vi "从数据库获取数据通用可配置(子VI).vi"(8 "错误输入（无错误）":errorcluster, 9 "查询参数数组":string[](array[string])=["CODMn", "CODCr", "DO", "铜", "PH", "氨氮", "比电导率", "水温", "COD", "浊度", "总氮", "总磷", "叶绿素a", "藻密度", "水位", "流速", "瞬时流量", "累积流量", "亚硝酸盐", "硫化物", "ORP", "铅", "镉", "锌", "镍", "锰", "汞"], 10 "table输入":string="实时数据") -> (0 "错误输出":errorcluster, 3 "簇数组":cluster{"待发送数据":string[][]}[][](array[cluster]))   [LabVIEW 2016, in "数据传输系统-02.lvlib"]
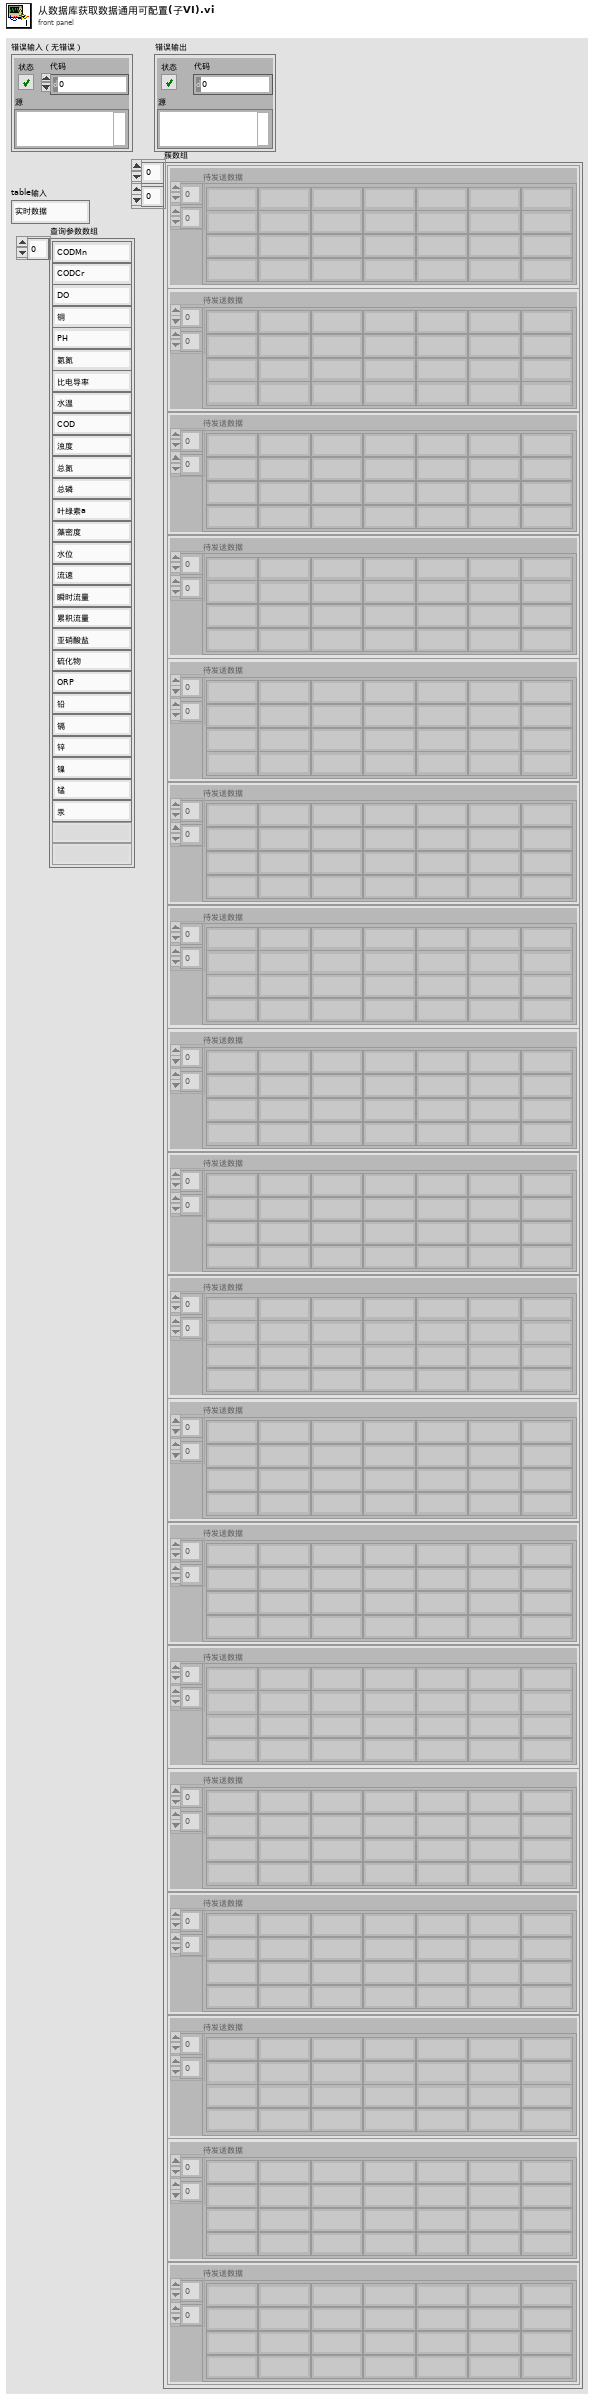
[diagram p1: front panel]
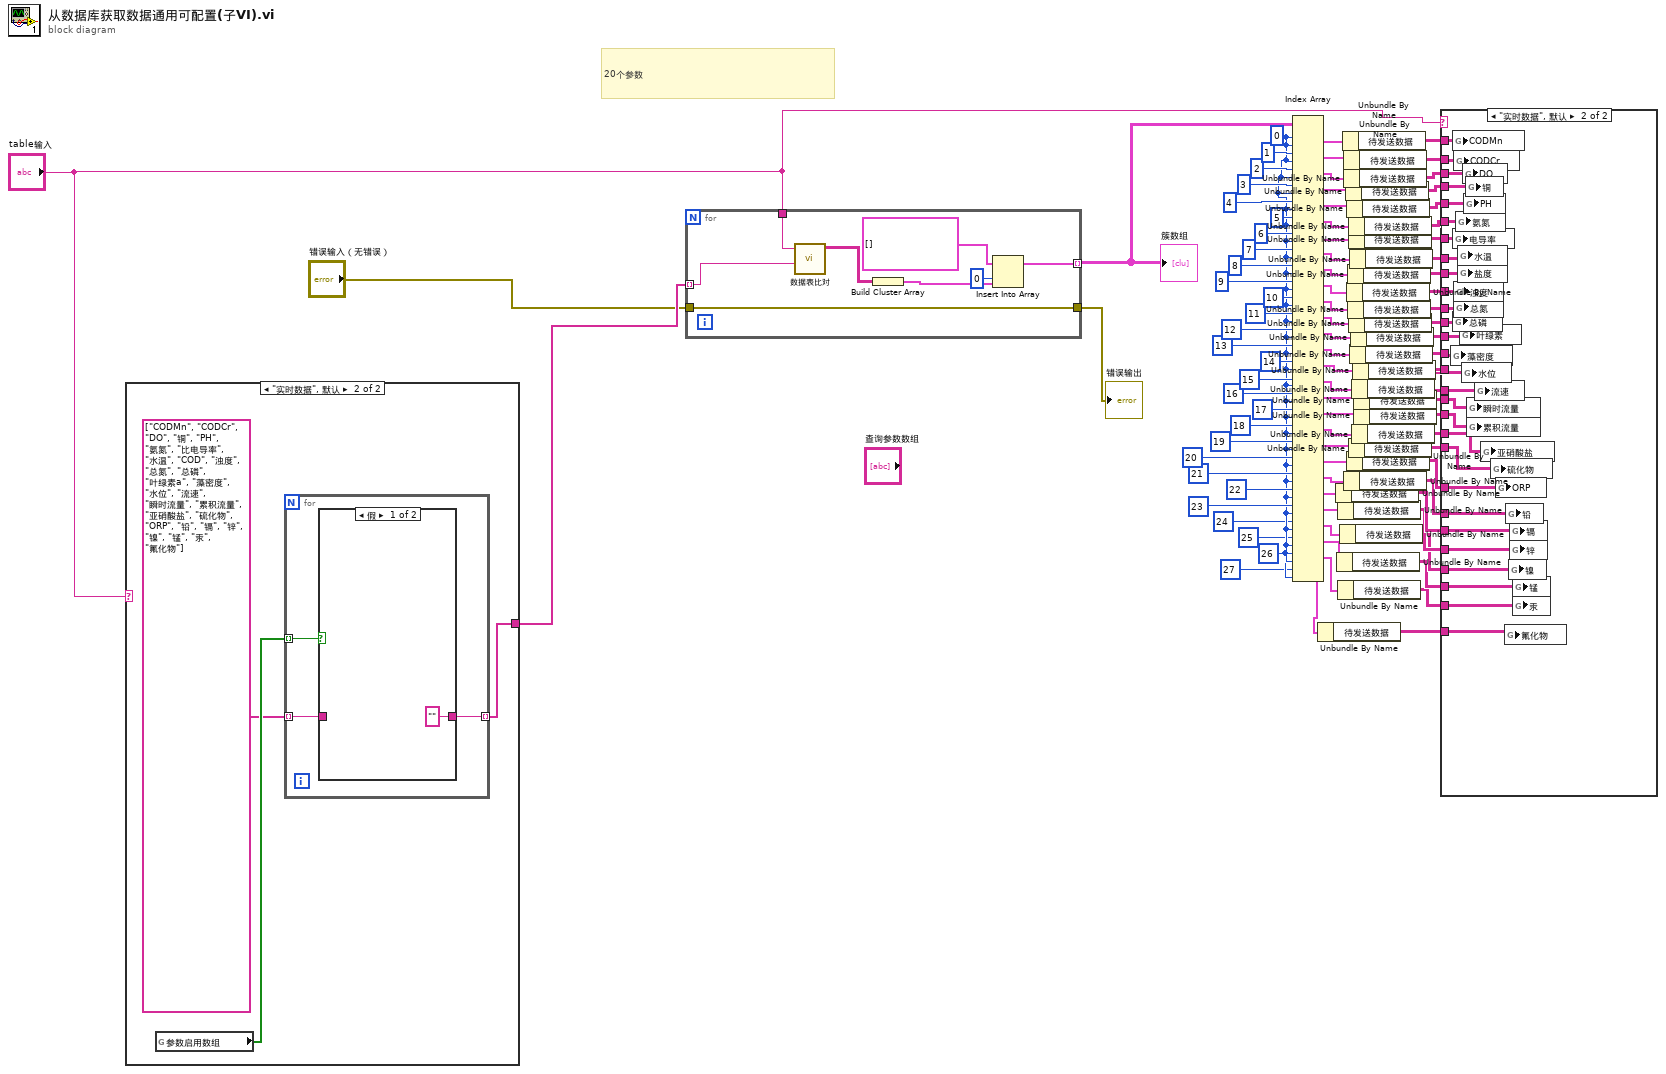
[diagram p0: block diagram]
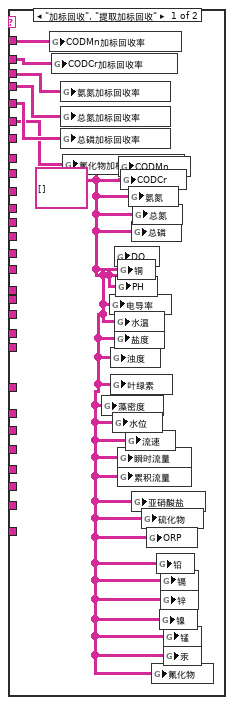
[diagram p2: hidden frame]
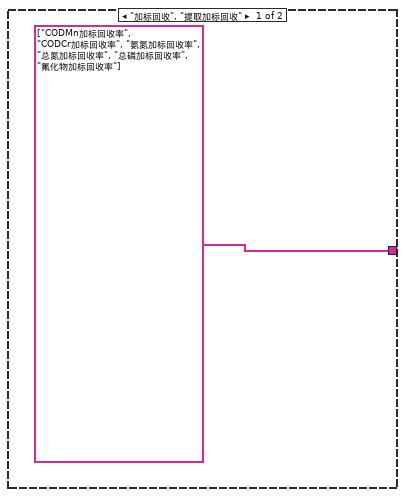
[diagram p3: hidden frame]
diagram:
  w4 = 26 ("禁用的索引 (行)")
  w14 = 0 ("索引 (行)")
  # "20个参数"
  n1 = case shown="\"实时数据\", 默认" "table输入" {
    tunnel: [string[] ["CODMn加标回收率", "CODCr加标回收率", "氨氮加标回收率", "总氮加标回收率", "总磷加标回收率", "氟化物加标回收率"] ("查询参数数组") w91] -> w46
    frame "加标回收", "提取加标回收" {
    }
    frame "实时数据", Default {
      n2 = global read "断电保存全局.vi" "参数启用数组"() -> (w93:bool[])
      n3 = for {
        tunnel: w93 -> [w96] mode=indexing
        tunnel: string[] ["CODMn", "CODCr", "DO", "铜", "PH", "氨氮", "比电导率", "水温", "COD", "浊度", "总氮", "总磷", "叶绿素a", "藻密度", "水位", "流速", "瞬时流量", "累积流量", "亚硝酸盐", "硫化物", "ORP", "铅", "镉", "锌", "镍", "锰", "汞", "氟化物"] ("数组") -> [w95] mode=indexing
        tunnel: [w94] -> w91 mode=indexing
        n4 = case shown="假" w96 {
          tunnel: ["" w98] -> w94
          tunnel: w95 -> [_ w98]
          frame False {
          }
          frame True {
          }
        }
      }
    }
  }
  n5 = for {
    tunnel: w46 -> [w100] mode=indexing
    tunnel: [w104] -> w88 mode=indexing
    tunnel: "table输入" -> [w101]
    tunnel: [w99] -> w89
    tunnel: "错误输入（无错误）" -> [w99]
    n6 = call "数据表比对.vi"("查询元素输入"=w100, "table输入"=w101) -> ("待发送数据"=w106:string[][])  [unwired: 6 in, 3 out]
    n7 = Build Cluster Array(w106) -> (w105:cluster{"待发送数据":string[][]}[])
    n8 = Insert Into Array(array=cluster{"待发送数据":string[][]}[] [] ("簇数组"), index=0 ("索引"), new element=w105) -> (w104:cluster{"待发送数据":string[][]}[])
  }
  "簇数组" <- w88
  "错误输出" <- w89
  n9 = Index Array(array=w88, index (row) #1=w14, index (col) #1=w14, index (row) #2=1 ("索引 (行)"), index (col) #2=w14, index (row) #3=2 ("索引 (行)"), index (col) #3=w14, index (row) #4=3 ("索引 (行)"), index (col) #4=w14, index (row) #5=4 ("索引 (行)"), index (col) #5=w14, index (row) #6=5 ("索引 (行)"), index (col) #6=w14, index (row) #7=6 ("索引 (行)"), index (col) #7=w14, index (row) #8=7 ("索引 (行)"), index (col) #8=w14, index (row) #9=8 ("索引 (行)"), index (col) #9=w14, index (row) #10=9 ("索引 (行)"), index (col) #10=w14, index (row) #11=10 ("索引 (行)"), index (col) #11=w14, index (row) #12=11 ("索引 (行)"), index (col) #12=w14, index (row) #13=12 ("索引 (行)"), index (col) #13=w14, index (row) #14=13 ("索引 (行)"), index (col) #14=w14, index (row) #15=14 ("禁用的索引 (行)"), index (col) #15=w14, index (row) #16=15 ("禁用的索引 (行)"), index (col) #16=w14, index (row) #17=16 ("禁用的索引 (行)"), index (col) #17=w14, index (row) #18=17 ("禁用的索引 (行)"), index (col) #18=w14, index (row) #19=18 ("禁用的索引 (行)"), index (col) #19=w14, index (row) #20=19 ("禁用的索引 (行)"), index (col) #20=w14, index (row) #21=20 ("禁用的索引 (行)"), index (col) #21=w14, index (row) #22=21 ("禁用的索引 (行)"), index (col) #22=w14, index (row) #23=22 ("禁用的索引 (行)"), index (col) #23=w14, index (row) #24=23 ("禁用的索引 (行)"), index (col) #24=w14, index (row) #25=24 ("禁用的索引 (行)"), index (col) #25=w14, index (row) #26=25 ("禁用的索引 (行)"), index (col) #26=w14, index (row) #27=w4, index (col) #27=w14, index (row) #28=27 ("禁用的索引 (行)"), index (col) #28=w4) -> (element #1=w87:cluster{"待发送数据":string[][]}, element #2=w72:cluster{"待发送数据":string[][]}, element #3=w71:cluster{"待发送数据":string[][]}, element #4=w70:cluster{"待发送数据":string[][]}, element #5=w69:cluster{"待发送数据":string[][]}, element #6=w68:cluster{"待发送数据":string[][]}, element #7=w66:cluster{"待发送数据":string[][]}, element #8=w67:cluster{"待发送数据":string[][]}, element #9=w65:cluster{"待发送数据":string[][]}, element #10=w64:cluster{"待发送数据":string[][]}, element #11=w63:cluster{"待发送数据":string[][]}, element #12=w62:cluster{"待发送数据":string[][]}, element #13=w61:cluster{"待发送数据":string[][]}, element #14=w60:cluster{"待发送数据":string[][]}, element #15=w41:cluster{"待发送数据":string[][]}, element #16=w39:cluster{"待发送数据":string[][]}, element #17=w38:cluster{"待发送数据":string[][]}, element #18=w37:cluster{"待发送数据":string[][]}, element #19=w32:cluster{"待发送数据":string[][]}, element #20=w28:cluster{"待发送数据":string[][]}, element #21=w27:cluster{"待发送数据":string[][]}, element #22=w20:cluster{"待发送数据":string[][]}, element #23=w19:cluster{"待发送数据":string[][]}, element #24=w18:cluster{"待发送数据":string[][]}, element #25=w11:cluster{"待发送数据":string[][]}, element #26=w9:cluster{"待发送数据":string[][]}, element #27=w8:cluster{"待发送数据":string[][]}, element #28=w2:cluster{"待发送数据":string[][]})
  n10 = Unbundle By Name(w2) -> ("待发送数据"=w1:string[][])
  n11 = Unbundle By Name(w19) -> ("待发送数据"=w16:string[][])
  n12 = Unbundle By Name(w9) -> ("待发送数据"=w7:string[][])
  n13 = Unbundle By Name(w18) -> ("待发送数据"=w15:string[][])
  n14 = Unbundle By Name(w8) -> ("待发送数据"=w6:string[][])
  n15 = Unbundle By Name(w11) -> ("待发送数据"=w10:string[][])
  n16 = Unbundle By Name(w87) -> ("待发送数据"=w86:string[][])
  n17 = Unbundle By Name(w72) -> ("待发送数据"=w59:string[][])
  n18 = Unbundle By Name(w71) -> ("待发送数据"=w58:string[][])
  n19 = Unbundle By Name(w20) -> ("待发送数据"=w17:string[][])
  n20 = Unbundle By Name(w70) -> ("待发送数据"=w57:string[][])
  n21 = Unbundle By Name(w69) -> ("待发送数据"=w56:string[][])
  n22 = Unbundle By Name(w64) -> ("待发送数据"=w51:string[][])
  n23 = Unbundle By Name(w27) -> ("待发送数据"=w24:string[][])
  n24 = Unbundle By Name(w65) -> ("待发送数据"=w52:string[][])
  n25 = Unbundle By Name(w63) -> ("待发送数据"=w50:string[][])
  n26 = Unbundle By Name(w68) -> ("待发送数据"=w55:string[][])
  n27 = Unbundle By Name(w66) -> ("待发送数据"=w54:string[][])
  n28 = Unbundle By Name(w62) -> ("待发送数据"=w49:string[][])
  n29 = Unbundle By Name(w28) -> ("待发送数据"=w25:string[][])
  n30 = Unbundle By Name(w67) -> ("待发送数据"=w53:string[][])
  n31 = Unbundle By Name(w60) -> ("待发送数据"=w48:string[][])
  n32 = Unbundle By Name(w61) -> ("待发送数据"=w47:string[][])
  n33 = Unbundle By Name(w39) -> ("待发送数据"=w36:string[][])
  n34 = Unbundle By Name(w32) -> ("待发送数据"=w26:string[][])
  n35 = Unbundle By Name(w41) -> ("待发送数据"=w40:string[][])
  n36 = Unbundle By Name(w38) -> ("待发送数据"=w35:string[][])
  n37 = Unbundle By Name(w37) -> ("待发送数据"=w34:string[][])
  n38 = case shown="\"实时数据\", 默认" "table输入" {
    tunnel: w86 -> [w113 w141]
    tunnel: w59 -> [w112 w140]
    tunnel: w58 -> [w111 w139]
    tunnel: w57 -> [w110 w138]
    tunnel: w56 -> [w109 w137]
    tunnel: w55 -> [w108 w136]
    tunnel: w54 -> [_ w135]
    tunnel: w53 -> [_ w134]
    tunnel: w52 -> [_ w133]
    tunnel: w51 -> [_ w132]
    tunnel: w50 -> [_ w131]
    tunnel: w49 -> [_ w130]
    tunnel: w48 -> [_ w129]
    tunnel: w47 -> [_ w128]
    tunnel: w40 -> [_ w127]
    tunnel: w36 -> [_ w126]
    tunnel: w35 -> [_ w125]
    tunnel: w34 -> [_ w124]
    tunnel: w26 -> [_ w123]
    tunnel: w25 -> [_ w122]
    tunnel: w24 -> [_ w121]
    tunnel: w17 -> [_ w120]
    tunnel: w16 -> [_ w119]
    tunnel: w15 -> [_ w118]
    tunnel: w10 -> [_ w117]
    tunnel: w7 -> [_ w116]
    tunnel: w6 -> [_ w115]
    tunnel: w1 -> [_ w114]
    frame "加标回收", "提取加标回收" {
      w107 = string[][] [] ("DO")
      n39 = global write "全局 所有参数.vi" "CODMn加标回收率"(w113) -> ()
      n40 = global write "全局 所有参数.vi" "CODCr加标回收率"(w112) -> ()
      n41 = global write "全局 所有参数.vi" "氨氮加标回收率"(w111) -> ()
      n42 = global write "全局 所有参数.vi" "总氮加标回收率"(w110) -> ()
      n43 = global write "全局 所有参数.vi" "总磷加标回收率"(w109) -> ()
      n44 = global write "全局 所有参数.vi" "氟化物加标回收率"(w108) -> ()
      n45 = global write "全局 所有参数.vi" "藻密度"(w107) -> ()
      n46 = global write "全局 所有参数.vi" "电导率"(w107) -> ()
      n47 = global write "全局 所有参数.vi" "浊度"(w107) -> ()
      n48 = global write "全局 所有参数.vi" "叶绿素"(w107) -> ()
      n49 = global write "全局 所有参数.vi" "水位"(w107) -> ()
      n50 = global write "全局 所有参数.vi" "DO"(w107) -> ()
      n51 = global write "全局 所有参数.vi" "水温"(w107) -> ()
      n52 = global write "全局 所有参数.vi" "盐度"(w107) -> ()
      n53 = global write "全局 所有参数.vi" "PH"(w107) -> ()
      n54 = global write "全局 所有参数.vi" "铜"(w107) -> ()
      n55 = global write "全局 所有参数.vi" "瞬时流量"(w107) -> ()
      n56 = global write "全局 所有参数.vi" "累积流量"(w107) -> ()
      n57 = global write "全局 所有参数.vi" "CODMn"(w107) -> ()
      n58 = global write "全局 所有参数.vi" "CODCr"(w107) -> ()
      n59 = global write "全局 所有参数.vi" "流速"(w107) -> ()
      n60 = global write "全局 所有参数.vi" "氨氮"(w107) -> ()
      n61 = global write "全局 所有参数.vi" "总磷"(w107) -> ()
      n62 = global write "全局 所有参数.vi" "亚硝酸盐"(w107) -> ()
      n63 = global write "全局 所有参数.vi" "总氮"(w107) -> ()
      n64 = global write "全局 所有参数.vi" "硫化物"(w107) -> ()
      n65 = global write "全局 所有参数.vi" "ORP"(w107) -> ()
      n66 = global write "全局 所有参数.vi" "氟化物"(w107) -> ()
      n67 = global write "全局 所有参数.vi" "铅"(w107) -> ()
      n68 = global write "全局 所有参数.vi" "镍"(w107) -> ()
      n69 = global write "全局 所有参数.vi" "镉"(w107) -> ()
      n70 = global write "全局 所有参数.vi" "锌"(w107) -> ()
      n71 = global write "全局 所有参数.vi" "锰"(w107) -> ()
      n72 = global write "全局 所有参数.vi" "汞"(w107) -> ()
    }
    frame "实时数据", Default {
      n73 = global write "全局 所有参数.vi" "藻密度"(w129) -> ()
      n74 = global write "全局 所有参数.vi" "CODMn"(w141) -> ()
      n75 = global write "全局 所有参数.vi" "电导率"(w135) -> ()
      n76 = global write "全局 所有参数.vi" "总磷"(w130) -> ()
      n77 = global write "全局 所有参数.vi" "CODCr"(w140) -> ()
      n78 = global write "全局 所有参数.vi" "浊度"(w132) -> ()
      n79 = global write "全局 所有参数.vi" "总氮"(w131) -> ()
      n80 = global write "全局 所有参数.vi" "氨氮"(w136) -> ()
      n81 = global write "全局 所有参数.vi" "水温"(w134) -> ()
      n82 = global write "全局 所有参数.vi" "盐度"(w133) -> ()
      n83 = global write "全局 所有参数.vi" "叶绿素"(w128) -> ()
      n84 = global write "全局 所有参数.vi" "水位"(w127) -> ()
      n85 = global write "全局 所有参数.vi" "DO"(w139) -> ()
      n86 = global write "全局 所有参数.vi" "PH"(w137) -> ()
      n87 = global write "全局 所有参数.vi" "铜"(w138) -> ()
      n88 = global write "全局 所有参数.vi" "瞬时流量"(w125) -> ()
      n89 = global write "全局 所有参数.vi" "累积流量"(w124) -> ()
      n90 = global write "全局 所有参数.vi" "流速"(w126) -> ()
      n91 = global write "全局 所有参数.vi" "亚硝酸盐"(w123) -> ()
      n92 = global write "全局 所有参数.vi" "硫化物"(w122) -> ()
      n93 = global write "全局 所有参数.vi" "ORP"(w121) -> ()
      n94 = global write "全局 所有参数.vi" "氟化物"(w114) -> ()
      n95 = global write "全局 所有参数.vi" "铅"(w120) -> ()
      n96 = global write "全局 所有参数.vi" "镍"(w117) -> ()
      n97 = global write "全局 所有参数.vi" "镉"(w119) -> ()
      n98 = global write "全局 所有参数.vi" "锌"(w118) -> ()
      n99 = global write "全局 所有参数.vi" "锰"(w116) -> ()
      n100 = global write "全局 所有参数.vi" "汞"(w115) -> ()
    }
  }
